vi "Receive Datagram.vi"(8 "error in (no error)":errorcluster, 10 "transfer group id":i32, 11 "UDPlog Transceiver in":refnum<class "UDPlog Transceiver.lvclass">) -> (0 "error out":errorcluster, 1 "transfer data":string, 2 "transfer id":i32, 3 "UDPlog Transceiver out":refnum<class "UDPlog Transceiver.lvclass">, 4 "valid":bool)   [LabVIEW 2023, in "UDPlog.lvlib" / "UDPlog Transceiver.lvclass"]
uses:
  UDPlog Transceiver.lvclass
  UDPlog Transceiver.lvclass/UDPlog Transceiver.ctl
  <vilib>/Utility/error.llb/Clear Errors.vi
  <vilib>/Utility/SystemLogging/Write to System Log.vi
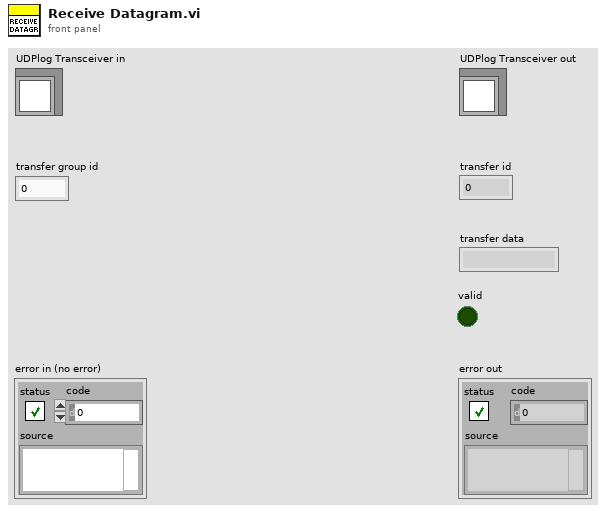
[diagram p1: front panel]
types:
  T1 = typedef "UDPlog.lvlib/UDPlog Transceiver.lvclass/Trasfer Group Parameters.ctl" = cluster{"transfers":T2[], "max size":i32, "timeout":i32}
  T2 = typedef "UDPlog.lvlib/UDPlog Transceiver.lvclass/Transfer Parameters.ctl" = cluster{"group offset":u64, "size":u64, "address":u32, "port":u16}
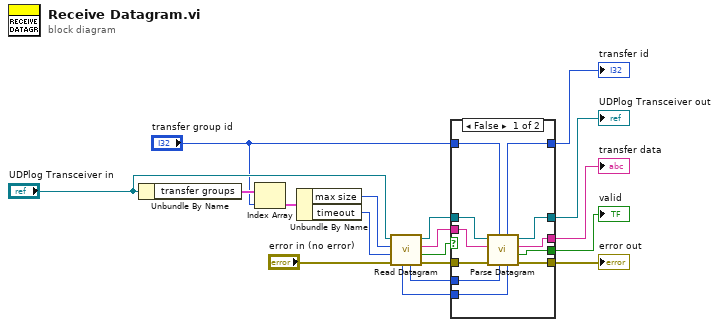
[diagram p0: block diagram]
diagram:
  n1 = Unbundle By Name("UDPlog Transceiver in") -> ("transfer groups"=w16:T1[])
  n2 = Index Array(array=w16, index="transfer group id") -> (element=w15:T1)
  n3 = Unbundle By Name(w15) -> ("max size"=w14:i32, "timeout"=w13:i32)
  n4 = call "Read Datagram.vi"("error in (no error)"="error in (no error)", "timeout ms (25000)"=w13, "max size (548)"=w14, "UDPlog Transceiver in"="UDPlog Transceiver in") -> ("error out"=w11:errorcluster, "timed out?"=w12:bool, "data"=w9:string, "UDPlog Transceiver out"=w10:refnum<class "UDPlog Transceiver.lvclass">, "source port"=w3:u16, "source address"=w2:u32)  [unwired: 2 in]
  n5 = case shown="False" w12 {
    tunnel: w11 -> [w29 w30]
    tunnel: w10 -> [w28 w31]
    tunnel: w9 -> [w27 _]
    tunnel: "transfer group id" -> [w26 _]
    tunnel: [w25 _] -> w7
    tunnel: [w24 _] -> w6
    tunnel: [w23 _] -> w5
    tunnel: [w22 w30] -> w4
    tunnel: w3 -> [w21 _]
    tunnel: w2 -> [w20 _]
    tunnel: [w19 w31] -> w1
    frame False {
      n6 = call-dynamic "Parse Datagram.vi"("source address"=w20, "source port"=w21, "transfer group id"=w26, "error in (no error)"=w29, "datagram"=w27, "UDPlog Transceiver in"=w28) -> ("error out"=w22:errorcluster, "valid"=w23:bool, "transfer data"=w24:string, "UDPlog Transceiver out"=w19:refnum<class "UDPlog Transceiver.lvclass">, "transfer id"=w25:i32)  [unwired: 1 in]
    }
    frame True {
    }
  }
  "error out" <- w4
  "UDPlog Transceiver out" <- w1
  "transfer id" <- w7
  "transfer data" <- w6
  "valid" <- w5
